vi "RequestOverride.vi"(8 "Error in":errorcluster[](array[cluster]), 11 "Visualize":refnum<class "VisualizePMU_class.lvclass">) -> (0 "Error out":errorcluster[](array[cluster]), 3 "RequestEvents":T1)   [LabVIEW 2014, in "Visualization.lvlib" / "VisualizePMU_class.lvclass"]
uses:
  VisualizePMU_class.lvclass
  VisializeBase_class/Requests/clRequestEvents.ctl
  VisializeBase_class/Requests/clUserEventType.ctl
  VisializeBase_class/VisualizeBase_class.lvclass
panel:
  # "This dynamic terminal makes the vi overridable and is marked in the base class as \"Must Override\".  \n\nSo any child class derived from this parent class must override this VI"
  # "If you want to add other Request Events, open this typedef, copy an existing event and rename it to your event name."
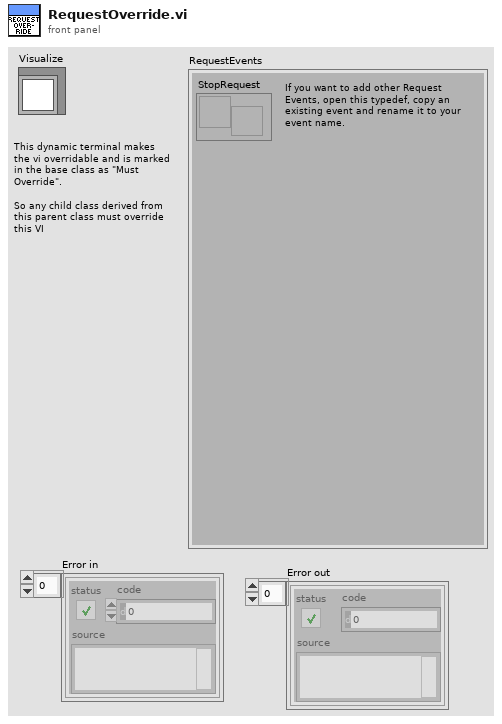
[diagram p1: front panel]
types:
  T1 = typedef "Visualization.lvlib/VisualizeBase_class.lvclass/clRequestEvents.ctl" = cluster{"StopRequest":refnum<user-event>}
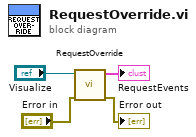
[diagram p0: block diagram]
diagram:
  n1 = call-parent "RequestOverride.vi"("Error in"="Error in", "Visualize"="Visualize") -> ("Error out"=→"Error out":errorcluster[], "RequestEvents"=→"RequestEvents":T1)  [unwired: 8 in]
